vi "Update Form.vi"(8 "error in (no error)":errorcluster, 9 "Table":refnum<class "Basic Table.lvclass">, 10 "Form ID":T1, 11 "Form Server in":refnum<class "Form Server.lvclass">) -> (0 "error out":errorcluster, 3 "Form Server out":refnum<class "Form Server.lvclass">)   [LabVIEW 2020, in "Form Server.lvlib" / "Form Server.lvclass"]
uses:
  Form Server.lvclass
  Autoclose manager/Form ID.ctl
  Database OOP/Table Libraries/Basic Table/Basic Table Class/Basic Table.lvclass
  Form Server.lvclass/Form Server.ctl
  Forms Model/Form Model Interfaces/Form Model Messages Messages/Update Table Msg/Update Table Msg.lvclass/Update Table Msg.ctl
  <vilib>/ActorFramework/Message Enqueuer/Message Enqueuer.lvclass/Message Enqueuer.ctl
  <vilib>/ActorFramework/Message Enqueuer/Enqueue.vi
  Forms Model/Form Model Interfaces/Form Model Messages Messages/Update Table Msg/Update Table Msg.lvclass
  C:/Program Files (x86)/National Instruments/LabVIEW 2020/vi.lib/ActorFramework/Message/Message.lvclass
  <vilib>/ActorFramework/Message Priority Queue/Priority Enqueue.vi
  Form Server Interfaces.lvlib
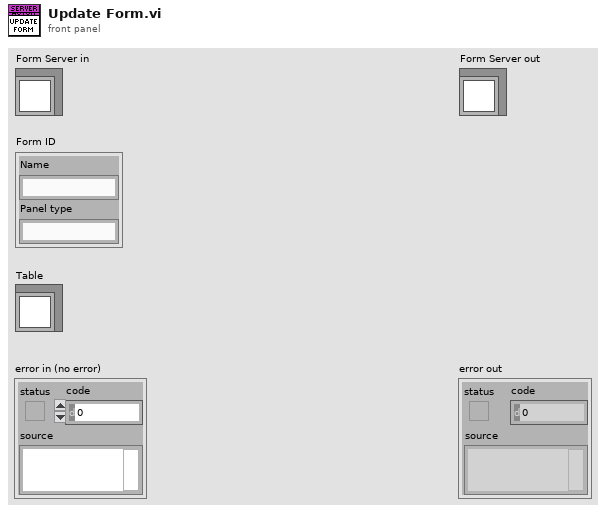
[diagram p1: front panel]
types:
  T1 = typedef "Form Server Interfaces.lvlib/Form ID.ctl" = cluster{"Name":string, "Panel type":string}
  T2 = map{T1, refnum<class "Message Enqueuer.lvclass">}
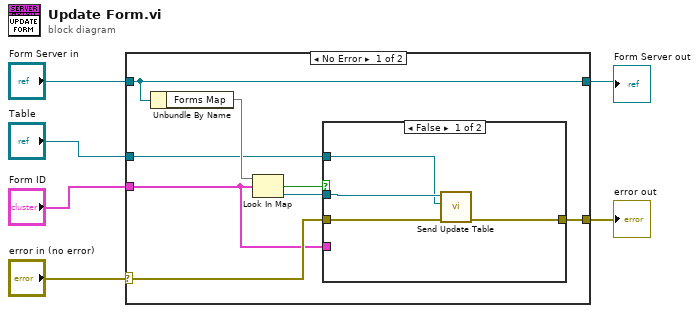
[diagram p0: block diagram]
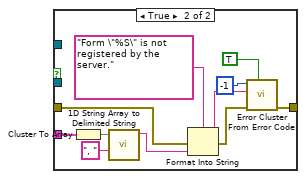
[diagram p2: hidden frame]
diagram:
  n1 = case shown="No Error" "error in (no error)" {
    selector: "error in (no error)" -> [w10 w31]
    tunnel: [w9 w31] -> w1
    tunnel: "Form Server in" -> [w14 w30]
    tunnel: [w14 w30] -> w4
    tunnel: "Form ID" -> [w8 _]
    tunnel: "Table" -> [w7 _]
    frame No Error {
      n2 = Unbundle By Name(w14) -> ("Forms Map"=w13:T2)
      n3 = Look In Map(map=w13, key=w8) -> (key not found?=w12:bool, value=w11:refnum<class "Message Enqueuer.lvclass">)  [unwired: 1 in]
      n4 = case shown="False" w12 {
        tunnel: w11 -> [w18 _]
        tunnel: w10 -> [w17 w24]
        tunnel: [w16 w23] -> w9
        tunnel: w8 -> [_ w29]
        tunnel: w7 -> [w15 _]
        frame False {
          n5 = call "Send Update Table.vi"("error in (no error)"=w17, "Table"=w15, "Message Enqueuer"=w18) -> ("error out"=w16:errorcluster)  [unwired: 7 in, 1 out]
        }
        frame True {
          n6 = Cluster To Array(cluster=w29) -> (array=w28:string[])
          n7 = call <vilib>:"1D String Array to Delimited String.vi"("delimiter"=", ", "string array"=w28) -> ("delimited string"=w25:string)  [unwired: 9 in]
          n8 = Format Into String(format string="Form \"%S\" is not registered by the server.", error in=w24, w25) -> (resulting string=w19:string, error out=w22:errorcluster)  [unwired: 1 in]
          n9 = call <vilib>:"Error Cluster From Error Code.vi"("show call chain? (False)"=TRUE, "error in (no error)"=w22, "error message (\"\")"=w19, "error code (0)"=-1 ("error code (no error:0)")) -> ("error out"=w23:errorcluster)  [unwired: 5 in]
        }
      }
    }
    frame Error {
    }
  }
  "error out" <- w1
  "Form Server out" <- w4
